vi "Bytes At Serial Port.vi"(0 "port number":i32) -> (1 "byte count":u32, 2 "error code":i32)   [LabVIEW 2020]
doc: "Returns the number of bytes in the input buffer of the serial port indicated in <B>port number</B>."
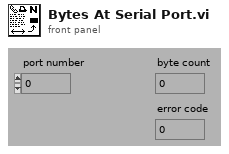
[diagram p1: front panel]
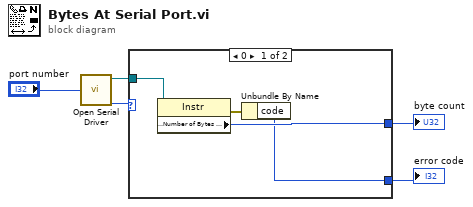
[diagram p0: block diagram]
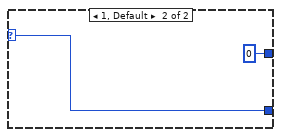
[diagram p2: hidden frame]
diagram:
  n1 = call "Open Serial Driver.vi"("port number"="port number") -> ("input refnum"=w4:refnum<visa-resource-name>, "output error"=w2:i32)  [unwired: 2 out]
  n2 = case shown="0" w2 {
    selector: w2 -> [_ w10]
    tunnel: w4 -> [w9 _]
    tunnel: [w8 u32 0 ("Bytes at Port")] -> w3
    tunnel: [w6 w10] -> w1
    frame 0 {
      n3 = property class="Instr"(reference=w9) -> (error out=w7:errorcluster, "Serial Settings:Number of Bytes at Serial Port"=w8:u32)  [unwired: 1 in, 1 out]
      n4 = Unbundle By Name(w7) -> ("code"=w6:i32)
    }
    frame 1, Default {
    }
  }
  "error code" <- w1
  "byte count" <- w3
